vi "AMWave.vi"() -> ()   [LabVIEW 2015]
panel:
  in  "Signal Frequency":i32
  in  "Sampling Frequency":i32
  out "AM Wave":cluster{dbl[], dbl[]}(graph)
  in  "Number of Samples":i32
  in  "Amplitude":i32
  in  "Modulation Frequency":i32
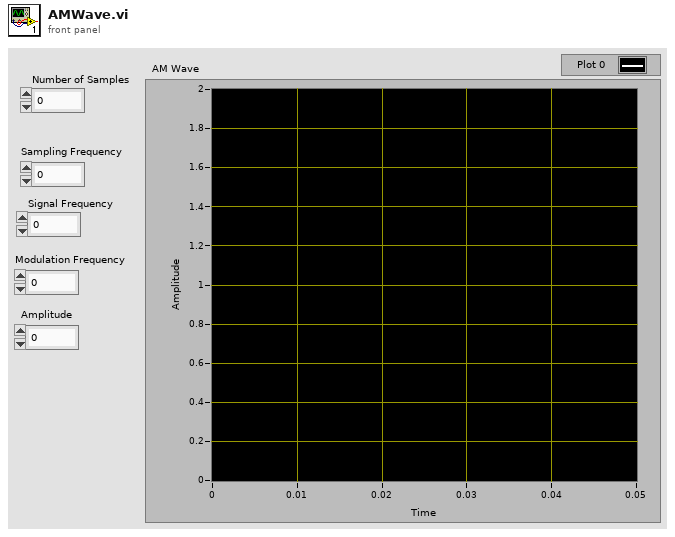
[diagram p1: front panel]
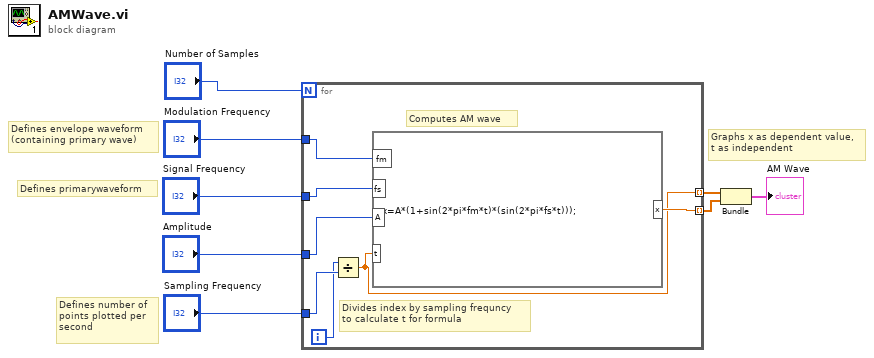
[diagram p0: block diagram]
diagram:
  # "Graphs x as dependent value,\nt as independent"
  # "Defines envelope waveform\n(containing primary wave)"
  # "Defines primarywaveform"
  # "Defines number of\npoints plotted per \nsecond"
  n1 = for {
    N: "Number of Samples" -> [_]
    tunnel: "Modulation Frequency" -> [w9]
    tunnel: "Amplitude" -> [w15]
    tunnel: [w14] -> w5 mode=indexing
    tunnel: [w12] -> w4 mode=indexing
    tunnel: "Sampling Frequency" -> [w13]
    tunnel: "Signal Frequency" -> [w10]
    i -> [w11]
    # "Divides index by sampling frequncy\nto calculate t for formula"
    # "Computes AM wave"
    n2 = Divide(x=w11, y=w13) -> (x/y=w12:dbl)
    n3 = formula code="x=A*(1+sin(2*pi*fm*t)*(sin(2*pi*fs*t)));"("fm"=w9, "t"=w12, "fs"=w10, "A"=w15) -> ("x"=w14:dbl)
  }
  n4 = Bundle(w4, w5) -> (→"AM Wave":cluster{dbl[], dbl[]})  [unwired: 1 in]
